vi "map_tool_to_subsystem-test.vi"() -> ()   [LabVIEW 2017, in "labview-standard-library.lvlib" / "automode-scripting.lvlib"]
uses:
  automode-scripting.lvlib
  type-defs/tool-assignments.ctl
panel:
  out "All passing?":bool
  out "x = y?":bool[](array[boolean])
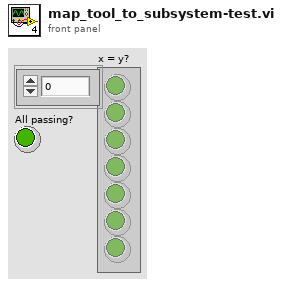
[diagram p1: front panel]
types:
  T1 = typedef "tool-assignments.ctl" = cluster{"Tool Name":string, "Subsystem":string, "Tool #":i32}[]
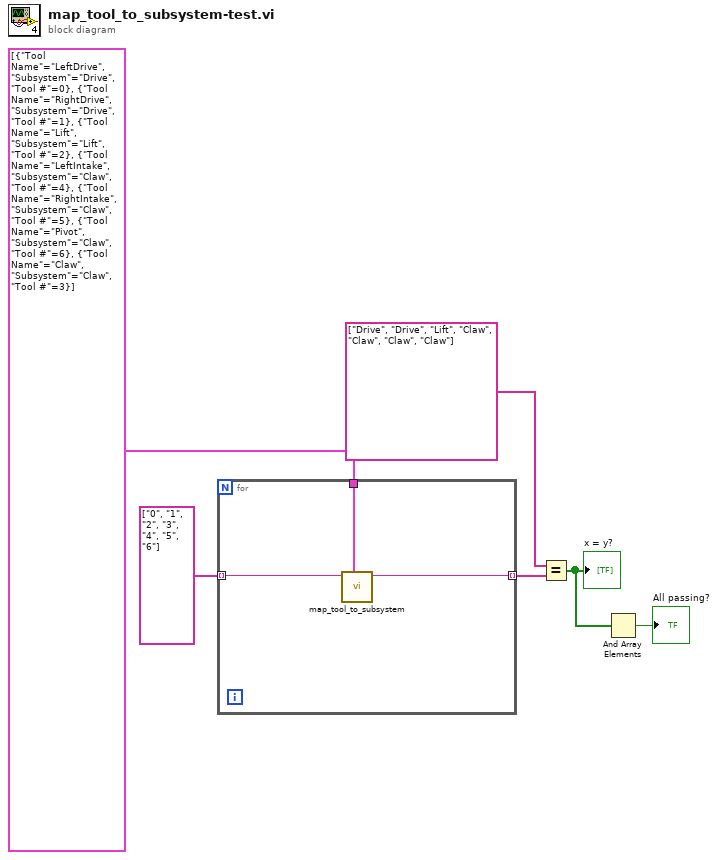
[diagram p0: block diagram]
diagram:
  n1 = for {
    tunnel: string[] ["0", "1", "2", "3", "4", "5", "6"] -> [w9] mode=indexing
    tunnel: T1 [{"Tool Name"="LeftDrive", "Subsystem"="Drive", "Tool #"=0}, {"Tool Name"="RightDrive", "Subsystem"="Drive", "Tool #"=1}, {"Tool Name"="Lift", "Subsystem"="Lift", "Tool #"=2}, {"Tool Name"="LeftIntake", "Subsystem"="Claw", "Tool #"=4}, {"Tool Name"="RightIntake", "Subsystem"="Claw", "Tool #"=5}, {"Tool Name"="Pivot", "Subsystem"="Claw", "Tool #"=6}, {"Tool Name"="Claw", "Subsystem"="Claw", "Tool #"=3}] ("Tool Assignments 2") -> [w8]
    tunnel: [w7] -> w3 mode=indexing
    n2 = call "map_tool_to_subsystem.vi"("Tool Assignments"=w8, "Tool #"=w9) -> ("Subsystem out"=w7:string)  [unwired: 9 in]
  }
  n3 = Equal?(x=string[] ["Drive", "Drive", "Lift", "Claw", "Claw", "Claw", "Claw"], y=w3) -> (x = y?=w2:bool[])
  "x = y?" <- w2
  n4 = And Array Elements(Boolean array=w2) -> (logical AND=→"All passing?":bool)
